vi "Draw Field XY Graph.vi"() -> (0 "XY Graph":cluster{"X":dbl, "Y":dbl}[](graph))   [LabVIEW 2014, in "Field.lvclass"]
uses:
  Field.lvclass
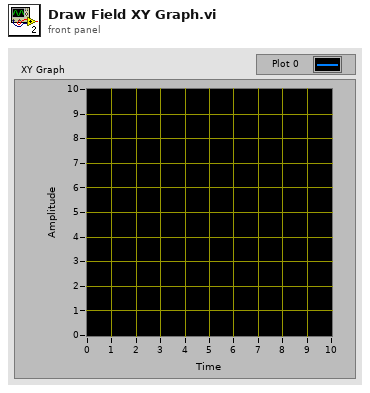
[diagram p1: front panel]
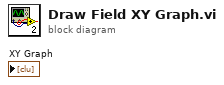
[diagram p0: block diagram]
diagram:
